vi "SelectRowTableCopy.vi"(8 "エラー入力":errorcluster, 9 "長さ":i32=1, 10 "指定行":i32, 11 "Tbl refnum":refnum<vi>) -> (0 "エラー出力":errorcluster, 2 "部分配列":string[][](array[string]), 3 "リファレンス出力":refnum<vi>)   [LabVIEW 2014]
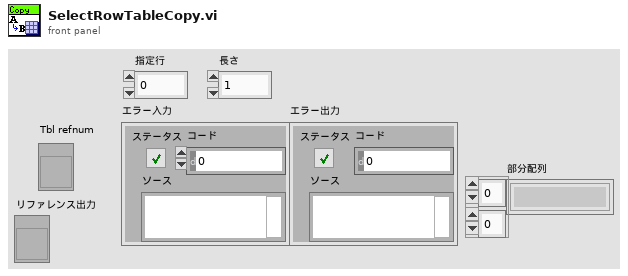
[diagram p1: front panel]
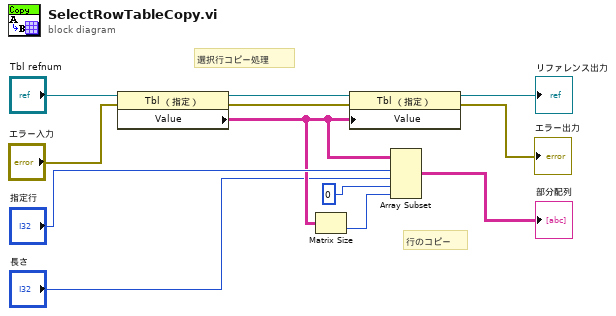
[diagram p0: block diagram]
diagram:
  # "行のコピー"
  # "選択行コピー処理"
  n1 = property class="Tbl （指定）"(reference="Tbl refnum", error in="エラー入力") -> (reference out=w8:refnum<vi>, error out=w7:errorcluster, "Value"=w5:string[][])
  n2 = Matrix Size(0:w5) -> (2:w2:i32)  [unwired: 1 out]
  n3 = property class="Tbl （指定）"(reference=w8, error in=w7, "Value"=w5) -> (reference out=→"リファレンス出力":refnum<vi>, error out=→"エラー出力":errorcluster)
  n4 = Array Subset(array=w5, index (row)="指定行", length (row)="長さ", index (col)=0 ("列1"), length (col)=w2) -> (→"部分配列":string[][])
